vi "Lead_2_ZPK.vi"(8 "error in (no error)":errorcluster, 11 "Lead params":T1={"f_lead [Hz]"=0.0, "alpha"=10.0}) -> (0 "error out":errorcluster, 3 "ZPK model":T2)   [LabVIEW 2020, in "PC-RT_Controller.lvlib"]
doc: "Convert lead with low-pass filter parameters (f_lead [Hz], alpha) into continuous time zero-pole-gain (ZPK) model."
uses:
  PC-RT_Controller.lvlib
  TypeDefs/ZPK_model.ctl
  TypeDefs/Lead params.ctl
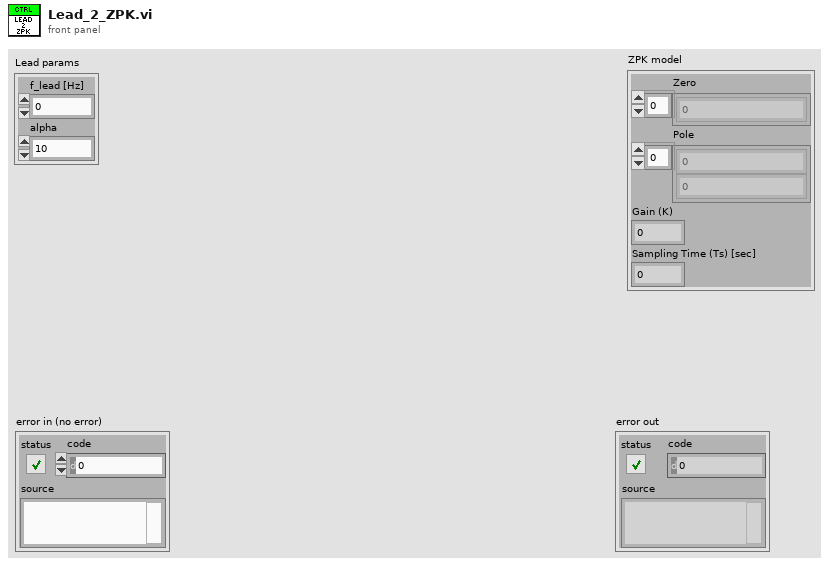
[diagram p1: front panel]
types:
  T1 = typedef "PC-RT_Controller.lvlib/Lead params.ctl" = cluster{"f_lead [Hz]":dbl, "alpha":dbl}
  T2 = typedef "PC-RT_Controller.lvlib/ZPK_model.ctl" = cluster{"Zero":cdb[], "Pole":cdb[], "Gain (K)":dbl, "Sampling Time (Ts) [sec]":dbl}
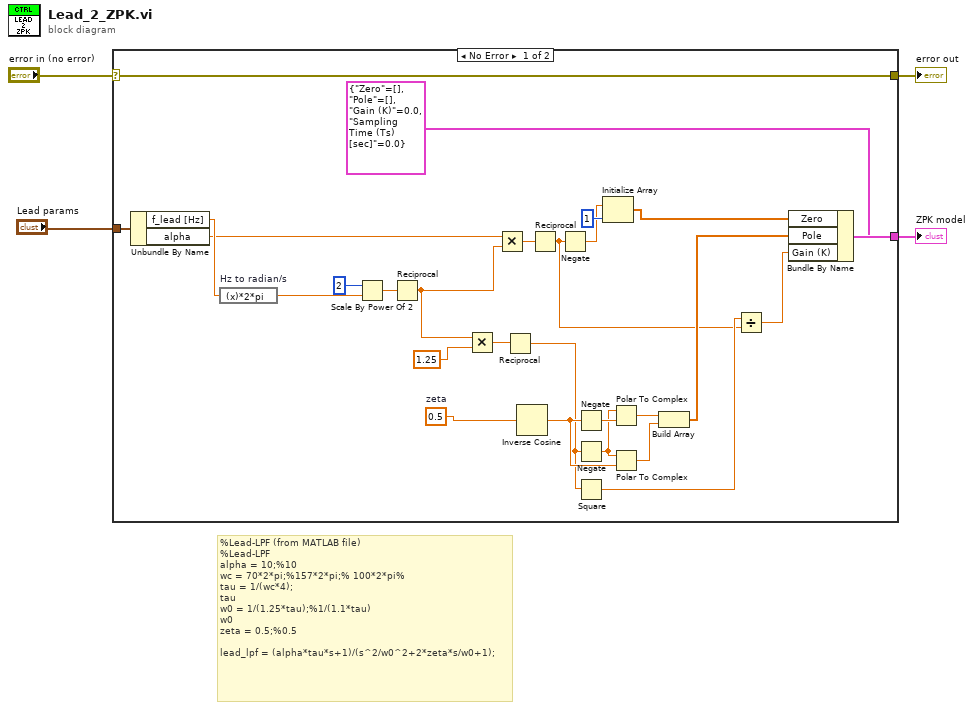
[diagram p0: block diagram]
diagram:
  # "%Lead-LPF (from MATLAB file)\n%Lead-LPF\nalpha = 10;%10\nwc = 70*2*pi;%157*2*pi;% 100*2*pi%\ntau = 1/(wc*4);\ntau\nw0 = 1/(1.25*tau);%1/(1.1*tau)\nw0\nzeta = 0.5;%0.5\n\nlead_lpf = (alpha*tau*s+1)/(s^2/w0^2+2*zeta*s/w0+1);"
  n1 = case shown="No Error" "error in (no error)" {
    selector: "error in (no error)" -> [w28 w32]
    tunnel: [w30 _] -> w4
    tunnel: "Lead params" -> [w29 _]
    tunnel: [w28 w32] -> w2
    frame No Error {
      w11 = 0.5  # zeta
      n2 = Unbundle By Name(w29) -> ("f_lead [Hz]"=w31:dbl, "alpha"=w23:dbl)
      n3 = expression code="(x)*2*pi" "Hz to radian/s"(w31) -> (w26:dbl)
      n4 = Scale By Power Of 2(n=i16 2, x=w26) -> (x*2^n=w24:dbl)
      n5 = Reciprocal(x=w24) -> (1/x=w19:dbl)
      n6 = Multiply(x=w19, y=1.25) -> (x*y=w17:dbl)
      n7 = Multiply(x=w23, y=w19) -> (x*y=w22:dbl)
      n8 = Reciprocal(x=w17) -> (1/x=w10:dbl)
      n9 = Inverse Cosine(1:w11) -> (0:w16:dbl)
      n10 = Reciprocal(x=w22) -> (1/x=w5:dbl)
      n11 = Negate(x=w5) -> (-x=w6:dbl)
      n12 = Negate(x=w16) -> (-x=w15:dbl)
      n13 = Negate(x=w10) -> (-x=w12:dbl)
      n14 = Square(x=w10) -> (x^2=w7:dbl)
      n15 = Initialize Array(w6, 1 ("dimension size")) -> (w20:dbl[])
      n16 = Polar To Complex(1:w15, 2:w12) -> (0:w13:cdb)
      n17 = Polar To Complex(1:w16, 2:w12) -> (0:w14:cdb)
      n18 = Build Array(w13, w14) -> (w9:cdb[])
      n19 = Divide(x=w7, y=w5) -> (x/y=w8:dbl)
      n20 = Bundle By Name(cluster=T2 {"Zero"=[], "Pole"=[], "Gain (K)"=0.0, "Sampling Time (Ts) [sec]"=0.0} ("ZPK model"), "Zero"=w20, "Pole"=w9, "Gain (K)"=w8) -> (w30:T2)
    }
    frame Error {
    }
  }
  "ZPK model" <- w4
  "error out" <- w2
